vi "test get elem of empty array.vi"() -> ()   [LabVIEW 2018, in "LV-Julia_ZMQ-Roundtrip_lib.lvlib"]
uses:
  LV-Julia_ZMQ-Roundtrip_lib.lvlib
panel:
  out "element":dbl
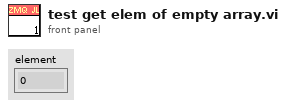
[diagram p1: front panel]
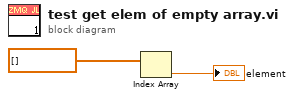
[diagram p0: block diagram]
diagram:
  n1 = Index Array(array=dbl[] [] ("Array")) -> (element=→"element":dbl)  [unwired: 1 in]
